vi "KGN Get Pump Mode.vi"(8 "Fehler (Eingang, kein Fehler)":errorcluster, 9 "Info Cluster":T4, 10 "VISA-Ressourcenname":refnum<visa-resource-name>, 11 "device (Eingang)":u32) -> (0 "Fehler (Ausgang)":errorcluster, 1 "Info Cluster out":T4, 2 "VISA-Ressourcenname out":refnum<visa-resource-name>, 3 "dup device (Ausgang)":u32, 4 "PumpMode-Cluster":T3(array[cluster]) {"concentratio mode" items=["water", "reagent"]; "Reagent" items=["HCl", "HF", "NH3", "HG", "PPM", "ORGANIC"]}, 6 "Kommandos gesendet":string)   [LabVIEW 2020, in "Linearisierung v2.lvlib" / "Gasteiler.lvlib" / "HovaCAL_Interface.lvlib" / "KGN.lvlib" / "KGN GUI Get.lvlib"]
uses:
  KGN GUI Get.lvlib
  Controls/Info Cluster.ctl
  Controls/Pump Concentration Mode.ctl
  Controls/Reagent.ctl
  get/get.lvlib
  Controls/Controls.lvlib
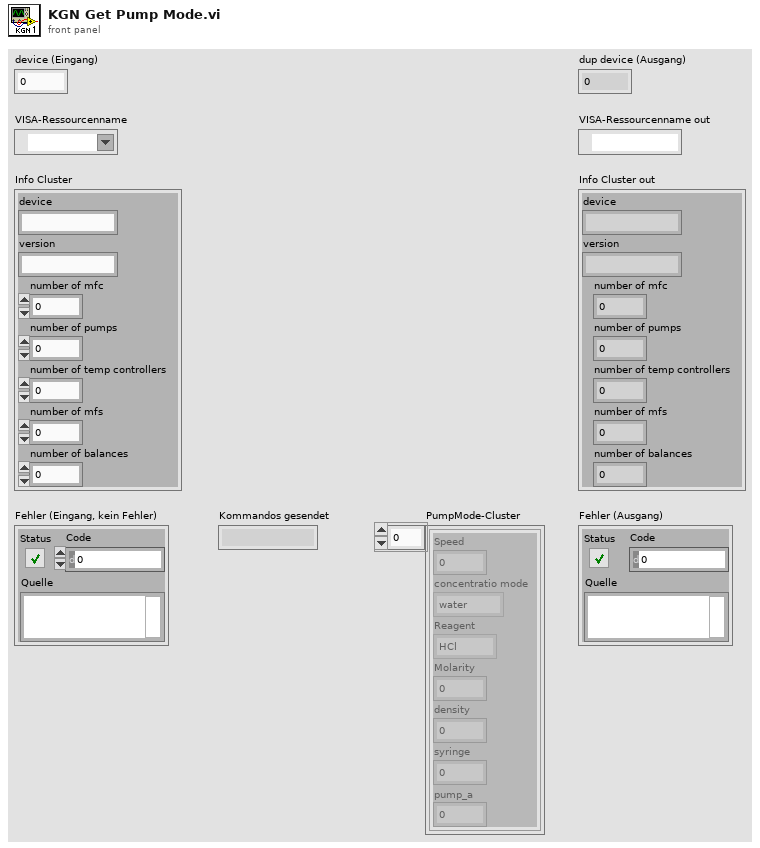
[diagram p1: front panel]
types:
  T1 = typedef "Linearisierung v2.lvlib/Gasteiler.lvlib/HovaCAL_Interface.lvlib/Controls.lvlib/Pump Concentration Mode.ctl" = i32
  T2 = typedef "Linearisierung v2.lvlib/Gasteiler.lvlib/HovaCAL_Interface.lvlib/Controls.lvlib/Reagent.ctl" = i32
  T3 = cluster{"Speed":dbl, "concentratio mode":T1, "Reagent":T2, "Molarity":dbl, "density":dbl, "syringe":dbl, "pump_a":dbl}[]
  T4 = typedef "Linearisierung v2.lvlib/Gasteiler.lvlib/HovaCAL_Interface.lvlib/Controls.lvlib/Info Cluster.ctl" = cluster{"device":string, "version":string, "number of mfc":i32, "number of pumps":i32, "number of temp controllers":i32, "number of mfs":i32, "number of balances":i32}
  T5 = cluster{"speed":dbl, "mode":dbl, "reagent":dbl, "molarity":dbl, "density":dbl, "syringe":dbl, "A":dbl}
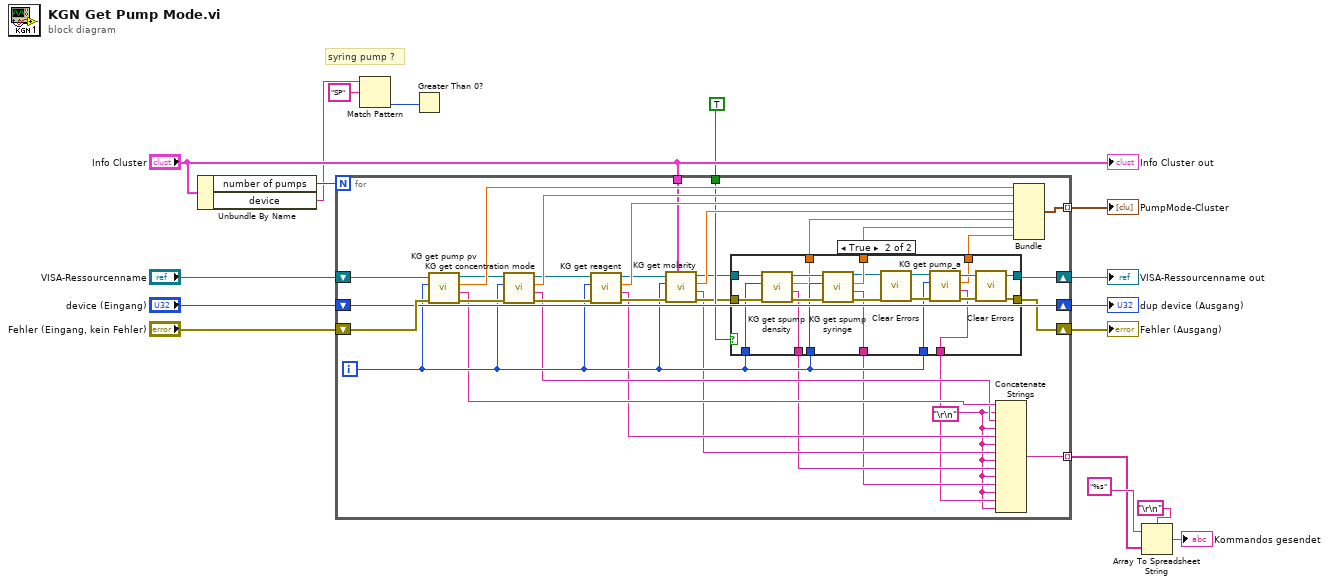
[diagram p0: block diagram]
diagram:
  # "syring pump ?"
  n1 = Unbundle By Name("Info Cluster") -> ("number of pumps"=w12:i32, "device"=w8:string)
  n2 = for {
    N: w12 -> [_]
    tunnel: [w46] -> w13 mode=indexing
    shift-right: [w45] -> w15
    shift-left: "device (Eingang)" -> [w45]
    shift-right: [w44] -> w14
    shift-left: "Fehler (Eingang, kein Fehler)" -> [w49]
    shift-right: [w41] -> w10
    shift-left: "VISA-Ressourcenname" -> [w42]
    tunnel: "Info Cluster" -> [w40]
    tunnel: TRUE -> [w37]
    tunnel: [w18] -> w2 mode=indexing
    i -> [w28]
    w19 = "\r\n"
    n3 = call "KG get pump pv.vi"("Fehler (Eingang, kein Fehler)"=w49, "pump"=w28, "VISA-Ressourcenname"=w42) -> ("Fehler (Ausgang)"=w35:errorcluster, "Kommando gesendet"=w26:string, "speed"=w50:dbl, "VISA-Ressourcenname (Ausgang)"=w36:refnum<visa-resource-name>)  [unwired: 5 in]
    n4 = call "KG get concentration mode.vi"("Fehler (Eingang, kein Fehler)"=w35, "pump"=w28, "VISA-Ressourcenname"=w36) -> ("Fehler (Ausgang)"=w33:errorcluster, "Kommando gesendet"=w25:string, "mode"=w48:dbl, "VISA-Ressourcenname (Ausgang)"=w34:refnum<visa-resource-name>)  [unwired: 5 in]
    n5 = call "KG get reagent.vi"("Fehler (Eingang, kein Fehler)"=w33, "pump"=w28, "VISA-Ressourcenname"=w34) -> ("Fehler (Ausgang)"=w31:errorcluster, "Kommando gesendet"=w24:string, "reagent"=w47:dbl, "VISA-Ressourcenname (Ausgang)"=w32:refnum<visa-resource-name>)  [unwired: 5 in]
    n6 = call "KG get molarity.vi"("Info Cluster"=w40, "Fehler (Eingang, kein Fehler)"=w31, "pump"=w28, "VISA-Ressourcenname"=w32) -> ("Fehler (Ausgang)"=w29:errorcluster, "Kommando gesendet"=w23:string, "molarity"=w43:dbl, "VISA-Ressourcenname (Ausgang)"=w30:refnum<visa-resource-name>)  [unwired: 4 in]
    n7 = case shown="True" w37 {
      tunnel: w30 -> [w52 w71]
      tunnel: w29 -> [w51 w70]
      tunnel: w28 -> [_ w69]
      tunnel: [w52 w61] -> w41
      tunnel: [w51 w58] -> w44
      tunnel: w28 -> [_ w66]
      tunnel: [_ w65] -> w39
      tunnel: [_ w64] -> w38
      tunnel: w28 -> [_ w57]
      tunnel: [_ w56] -> w27
      tunnel: [_ w55] -> w22
      tunnel: [_ w54] -> w21
      tunnel: [_ w53] -> w20
      frame False {
      }
      frame True {
        n8 = call "KG get spump density.vi"("Fehler (Eingang, kein Fehler)"=w70, "pump"=w69, "VISA-Ressourcenname"=w71) -> ("Fehler (Ausgang)"=w67:errorcluster, "Kommando gesendeet"=w55:string, "density"=w65:dbl, "VISA-Ressourcenname (Ausgang)"=w68:refnum<visa-resource-name>)  [unwired: 5 in]
        n9 = call "KG get spump syringe.vi"("Fehler (Eingang, kein Fehler)"=w67, "pump"=w66, "VISA-Ressourcenname"=w68) -> ("Fehler (Ausgang)"=w63:errorcluster, "Kommando gesendet"=w54:string, "syringe"=w64:dbl, "VISA-Ressourcenname (Ausgang)"=w62:refnum<visa-resource-name>)  [unwired: 5 in]
        n10 = call <vilib>:"Clear Errors.vi"("error in (no error)"=w63) -> ("error out"=w60:errorcluster)  [unwired: 5 in, 1 out]
        n11 = call "KG get pump_a.vi"("Fehler (Eingang, kein Fehler)"=w60, "pump"=w57, "VISA-Ressourcenname"=w62) -> ("Fehler (Ausgang)"=w59:errorcluster, "Kommando gesendet"=w53:string, "A"=w56:dbl, "VISA-Ressourcenname (Ausgang)"=w61:refnum<visa-resource-name>)  [unwired: 5 in]
        n12 = call <vilib>:"Clear Errors.vi"("error in (no error)"=w59) -> ("error out"=w58:errorcluster)  [unwired: 5 in, 1 out]
      }
    }
    n13 = Concatenate Strings(w26, w19, w25, w19, w24, w19, w23, w19, w22, w19, w21, w19, w20, w19) -> (w18:string)
    n14 = Bundle("speed"=w50, "mode"=w48, "reagent"=w47, "molarity"=w43, "density"=w39, "syringe"=w38, "A"=w27) -> (w46:T5)  [unwired: 1 in]
  }
  "dup device (Ausgang)" <- w15
  "Fehler (Ausgang)" <- w14
  "PumpMode-Cluster" <- w13
  "VISA-Ressourcenname out" <- w10
  n15 = Match Pattern(string=w8, regular expression="SP" ("Regulärer Ausdruck")) -> (offset past match=w6:i32)  [unwired: 1 in, 3 out]
  n16 = Greater Than 0?(x=w6) -> ()  [unwired: 1 out]
  n17 = Array To Spreadsheet String(delimiter (Tab)="\r\n", array=w2, 3:"%s" ("Format-String")) -> (spreadsheet string=→"Kommandos gesendet":string)
  "Info Cluster out" <- "Info Cluster"
